vi "outputs.vi"() -> ()   [LabVIEW 2018]
panel:
  out "Wheel_4_Azimuth_Current":dbl
  out "Wheel_2_Azimuth_Current":dbl
  out "Wheel_3_Azimuth_Current":dbl
  out "Wheel_1_Azimuth_Current":dbl
  out "Wheel_4_Azimuth_Goal":dbl
  out "Wheel_2_Azimuth_Goal":dbl
  out "Wheel_3_Azimuth_Goal":dbl
  out "Wheel_1_Azimuth_Goal":dbl
  out "Wheel_4_Power":dbl
  out "Wheel_2_Power":dbl
  out "Shifter_State":bool
  out "Butterfly_State":bool
  out "Wheel_3_Power":dbl
  out "Wheel_1_Power":dbl
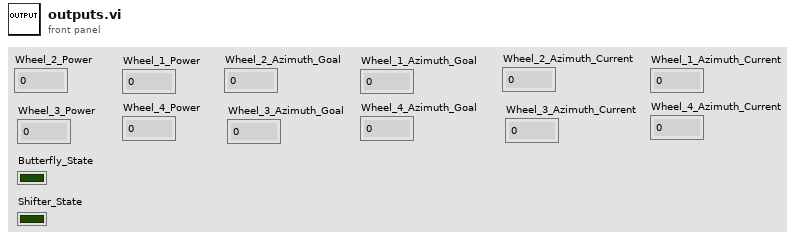
[diagram p1: front panel]
diagram:
